vi "Add Color Item.vi"(6 "Color Ramp Ref":refnum<vi>, 8 "error in (no error)":errorcluster, 9 "Numeric Ref Array In":refnum<vi>[](array[refnum]), 10 "Color Ref Array In":refnum<vi>[](array[refnum]), 11 "Slider Ref Array":refnum<vi>[](array[refnum])) -> (0 "error out":errorcluster, 5 "Slider Ref":refnum<vi>)   [LabVIEW 2020, in "3D Plot.lvclass"]
uses:
  <vilib>/Math Plots/3D Math Plots/3D Plot/3D Plot/3D Plot.lvclass
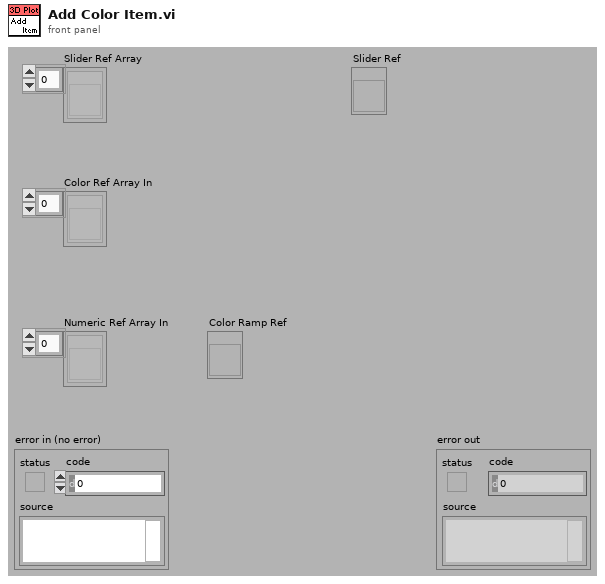
[diagram p1: front panel]
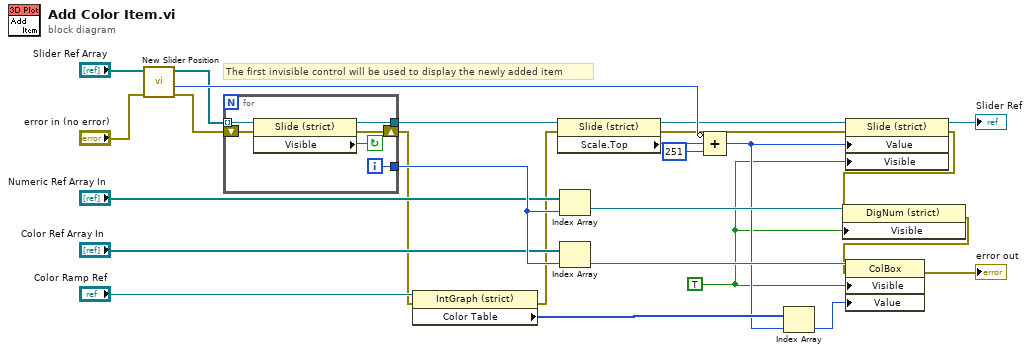
[diagram p0: block diagram]
diagram:
  w14 = TRUE ("Visible")
  # "The first invisible control will be used to display the newly added item"
  n1 = call <vilib>:"New Slider Position.vi"("error in (no error)"="error in (no error)", "Slider Ref Array"="Slider Ref Array") -> ("error out"=w2:errorcluster, "Vertical Position Out"=w23:i32, "Dup Slider Ref Array"=w1:refnum<vi>[])  [unwired: 7 out]
  n2 = for {
    tunnel: w1 -> [w32] mode=indexing
    tunnel: [w31] -> w17
    tunnel: [w30] -> w26
    shift-right: [w27] -> w10
    shift-left: w2 -> [w28]
    i -> [w31]
    stop <- w29 continue-if-true
    n3 = property class="Slide (strict)"(reference=w32, error in=w28) -> (reference out=w30:refnum<vi>, error out=w27:errorcluster, "Visible"=w29:bool)
  }
  n4 = property class="IntGraph (strict)"(reference="Color Ramp Ref", error in=w10) -> (error out=w9:errorcluster, "Color Table"=w18:u32[])  [unwired: 1 out]
  n5 = property class="Slide (strict)"(reference=w26, error in=w9) -> (reference out=w21:refnum<vi>, error out=w8:errorcluster, "Scale.Top"=w22:i32)
  n6 = Index Array(array="Numeric Ref Array In", index=w17) -> (element=w24:refnum<vi>)
  n7 = Index Array(array="Color Ref Array In", index=w17) -> (element=w25:refnum<vi>)
  n8 = Compound Arithmetic op=ADD(invert w23, w22, 251 ("value")) -> (w16:i32)
  n9 = Index Array(array=w18, index=w16) -> (element=w15:u32)
  n10 = property class="Slide (strict)"(reference=w21, error in=w8, "Value"=w16, "Visible"=w14) -> (reference out=→"Slider Ref":refnum<vi>, error out=w7:errorcluster)
  n11 = property class="DigNum (strict)"(reference=w24, error in=w7, "Visible"=w14) -> (error out=w6:errorcluster)  [unwired: 1 out]
  n12 = property class="ColBox"(reference=w25, error in=w6, "Visible"=w14, "Value"=w15) -> (error out=→"error out":errorcluster)  [unwired: 1 out]
